vi "题4.3.vi"() -> ()   [LabVIEW 2017]
panel:
  out "温度":string
  in  "停止":bool
  out "温度计":dbl(slide) scale=0.0..100.0
  in  "温度单位":bool
  # "°F"
  # "°C"
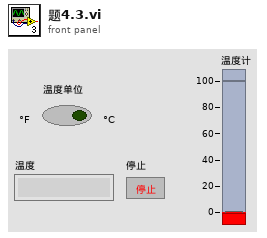
[diagram p1: front panel]
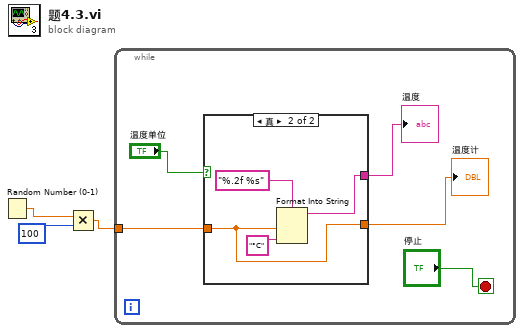
[diagram p0: block diagram]
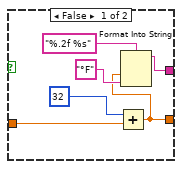
[diagram p2: hidden frame]
diagram:
  n1 = Random Number (0-1)() -> (number: 0 to 1=w3:dbl)
  n2 = Multiply(x=w3, y=100) -> (x*y=w1:dbl)
  n3 = while {
    tunnel: w1 -> [w6]
    stop <- "停止" stop-if-true
    n4 = case shown="真" "温度单位" {
      tunnel: [w11 w17] -> w5
      tunnel: w6 -> [w13 w16]
      tunnel: [w10 w16] -> w4
      frame False {
        n5 = Add(x=32, y=w13) -> (x+y=w10:dbl)
        n6 = Format Into String(format string="%.2f %s" ("格式字符串"), w10, "°F") -> (resulting string=w11:string)  [unwired: 2 in, 1 out]
      }
      frame True {
        n7 = Format Into String(format string="%.2f %s" ("格式字符串"), w16, "°C") -> (resulting string=w17:string)  [unwired: 2 in, 1 out]
      }
    }
    "温度计" <- w4
    "温度" <- w5
  }
